vi "stopSender.vi"(8 "error in (no error)":errorcluster, 11 "TcpServer in":refnum<class "TcpServer.lvclass">) -> (0 "error out":errorcluster, 3 "TcpServer out":refnum<class "TcpServer.lvclass">)   [LabVIEW 2018, in "TcpServer.lvclass"]
doc: "Send a signal to stop the Sender Loop (inside of readWritePacket.vi)"
uses:
  TcpServer.lvclass
  typedef/tcpPacketTypeDef.ctl
  TcpServer.lvclass/TcpServer.ctl
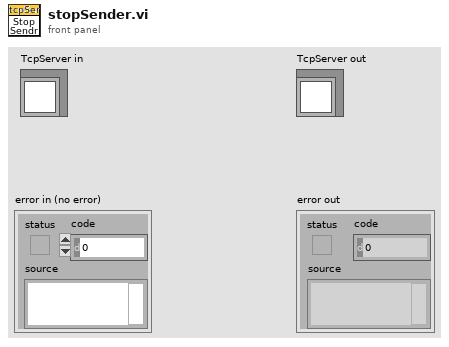
[diagram p1: front panel]
types:
  T1 = typedef "TcpServer.lvclass/tcpPacketTypeDef.ctl" = cluster{"packet":string, "firstPacket":bool, "firstConnection":bool}
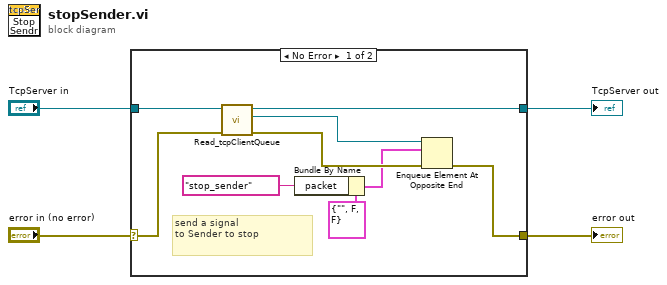
[diagram p0: block diagram]
diagram:
  n1 = case shown="No Error" "error in (no error)" {
    selector: "error in (no error)" -> [w9 w15]
    tunnel: [w8 w15] -> w3
    tunnel: [w11 w14] -> w1
    tunnel: "TcpServer in" -> [w12 w14]
    frame No Error {
      # "send a signal \nto Sender to stop"
      n2 = call "Read_tcpClientQueue.vi"("error in (no error)"=w9, "tcpServer in"=w12) -> ("error out"=w10:errorcluster, "tcpClientQueue"=w13:refnum<queue>, "tcpServer out"=w11:refnum<class "TcpServer.lvclass">)  [unwired: 7 in]
      n3 = Bundle By Name(cluster=T1 {"packet"="", "firstPacket"=FALSE, "firstConnection"=FALSE} ("packetConnID"), "packet"="stop_sender") -> (w5:T1)
      n4 = Enqueue Element At Opposite End(queue=w13, element=w5, error in (no error)=w10) -> (error out=w8:errorcluster)  [unwired: 1 in, 2 out]
    }
    frame Error {
    }
  }
  "error out" <- w3
  "TcpServer out" <- w1
